vi "SetEnumValueByString.vi"(8 "error in (no error)":errorcluster caption="错误输入（无错误）", 9 "strValue":string, 10 "strKey":string, 11 "handle":u64) -> (0 "error out":errorcluster caption="错误输出", 2 "function return":i32, 3 "handle out":u64)   [LabVIEW 2013, in "MvCameraControl.lvlib"]
doc: "MV_LV_API int __stdcall SetEnumValue( void* handle, const char* strValue, unsigned int nValue);"
uses:
  MvCameraControl.lvlib
  MvCameraControl.dll
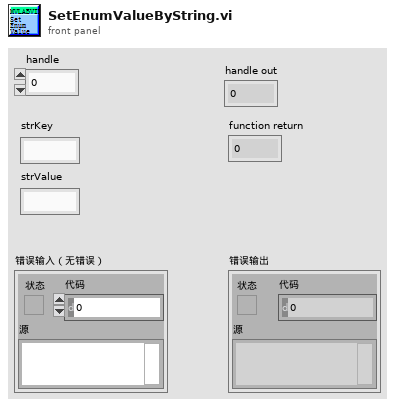
[diagram p1: front panel]
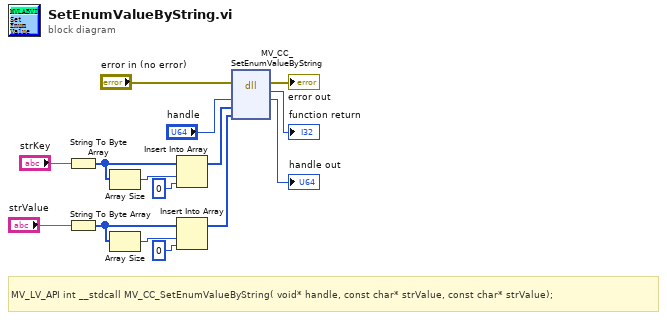
[diagram p0: block diagram]
diagram:
  # "MV_LV_API int __stdcall MV_CC_SetEnumValueByString( void* handle, const char* strValue, const char* strValue);"
  n1 = String To Byte Array(string="strKey") -> (unsigned byte array=w10:u8[])
  n2 = String To Byte Array(string="strValue") -> (unsigned byte array=w4:u8[])
  n3 = Array Size(array=w10) -> (size(s)=w9:i32)
  n4 = Array Size(array=w4) -> (size(s)=w3:i32)
  n5 = Insert Into Array(array=w10, index=w9, new element=u8 0 ("新元素/子数组")) -> (w7:u8[])
  n6 = Insert Into Array(array=w4, index=w3, new element=u8 0 ("新元素/子数组")) -> (w1:u8[])
  n7 = dll-call lib="MvCameraControl.dll" fn="MV_CC_SetEnumValueByString"(error in="error in (no error)", "handle"="handle", "strKey"=w7, "nValue"=w1) -> (error out=→"error out":errorcluster, "返回类型"=→"function return":i32, "handle"=→"handle out":u64)  [unwired: 4 in, 1 out]
